vi "Create Counter Driven Output Module.vi"(8 "error in":errorcluster, 9 "channel settings":T2[](array[typedef]), 10 "drive from slot":T1, 11 "module in":refnum<class "Module.lvclass">) -> (0 "error out":errorcluster, 3 "module out":refnum<class "Module.lvclass">)   [LabVIEW 2017, in "Scan Engine Scripting.lvlib" / "Module.lvclass"]
uses:
  Module.lvclass
  Mode Classes/Controls/counter driven output channel settings.ctl
  Channel Classes/Counter Driven Output Channel/Counter Driven State.ctl
  Mode Classes/Counter Driven Output Mode/Drive from Slot.ctl
  Mode Classes/Counter Driven Output Mode/Counter Driven Output Mode.lvclass
  C:/Users/nitest/Documents/niveristand-scan-engine-ethercat-custom-device/Custom Device Source/Scripting/Modules/Mode Classes/Mode/Mode.lvclass
  Channel Classes/Counter Driven Output Channel/Counter Driven Output Channel.lvclass
  C:/Users/nitest/Documents/niveristand-scan-engine-ethercat-custom-device/Custom Device Source/Scripting/Modules/Channel Classes/Channel/Channel.lvclass
  Scan Engine Scripting.lvlib
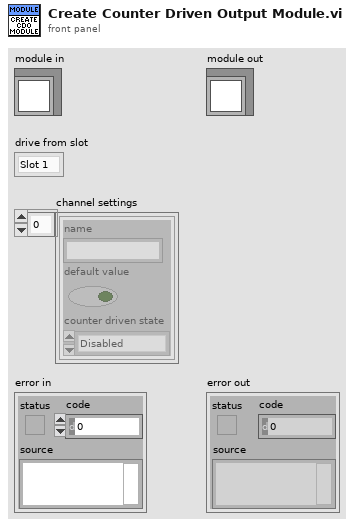
[diagram p1: front panel]
types:
  T1 = typedef "Scan Engine Scripting.lvlib/Counter Driven Output Mode.lvclass/Drive from Slot.ctl" = enum16{"Slot 1", "Slot 2", "Slot 3", "Slot 4", "Slot 5", "Slot 6", "Slot 7", "Slot 8"}
  T2 = typedef "Scan Engine Scripting.lvlib/counter driven output channel settings.ctl" = cluster{"name":string, "default value":bool, "counter driven state":T3}
  T3 = typedef "Scan Engine Scripting.lvlib/Counter Driven Output Channel.lvclass/Counter Driven State.ctl" = enum16{"Disabled", "Enabled"}
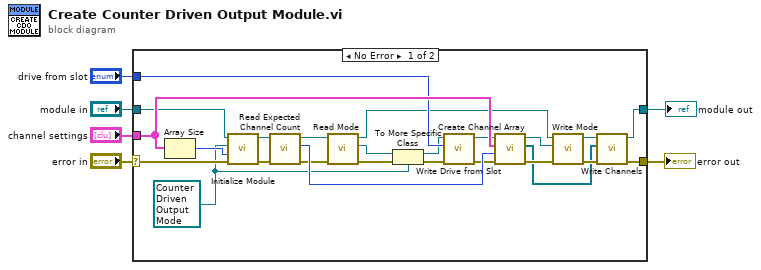
[diagram p0: block diagram]
diagram:
  n1 = case shown="No Error" "error in" {
    selector: "error in" -> [w30 w33]
    tunnel: [w7 w33] -> w1
    tunnel: [w27 w32] -> w2
    tunnel: "module in" -> [w25 w32]
    tunnel: "channel settings" -> [w28 _]
    tunnel: "drive from slot" -> [w24 _]
    frame No Error {
      w17 = refnum<class "Counter Driven Output Mode.lvclass"> refnum ("Scan Engine Scripting.lvlib:Counter Driven Output Mode.lvclass")
      n2 = Array Size(array=w28) -> (size(s)=w21:i32)
      n3 = call-dynamic "Initialize Module.vi"("error in"=w30, "channel array size"=w21, "mode"=w17, "module in"=w25) -> ("error out"=w31:errorcluster, "module out"=w29:refnum<class "Module.lvclass">)  [unwired: 6 in]
      n4 = call-dynamic "Read Expected Channel Count.vi"("error in"=w31, "module in"=w29) -> ("error out"=w20:errorcluster, "expected channel count"=w26:i32, "module out"=w9:refnum<class "Module.lvclass">)  [unwired: 7 in]
      n5 = call-dynamic "Read Mode.vi"("error in"=w20, "module in"=w9) -> ("error out"=w18:errorcluster, "mode"=w19:refnum<class "Mode.lvclass">, "module out"=w8:refnum<class "Module.lvclass">)  [unwired: 7 in]
      n6 = To More Specific Class(target class=w17, reference=w19, error in=w18) -> (specific class reference=w16:refnum<class "Counter Driven Output Mode.lvclass">, error out=w15:errorcluster)
      n7 = call-dynamic "Write Drive from Slot.vi"("error in"=w15, "drive from slot"=w24, "counter driven output mode in"=w16) -> ("error out"=w23:errorcluster, "counter driven output mode out"=w22:refnum<class "Counter Driven Output Mode.lvclass">)  [unwired: 7 in]
      n8 = call "Create Channel Array.vi"("error in"=w23, "array size"=w26, "channel settings"=w28, "counter driven output mode in"=w22) -> ("error out"=w12:errorcluster, "channels"=w10:refnum<class "Counter Driven Output Channel.lvclass">[], "counter driven output mode out"=w13:refnum<class "Counter Driven Output Mode.lvclass">)  [unwired: 5 in]
      n9 = call-dynamic "Write Mode.vi"("error in"=w12, "mode"=w13, "module in"=w8) -> ("error out"=w11:errorcluster, "module out"=w14:refnum<class "Module.lvclass">)  [unwired: 7 in]
      n10 = call-dynamic "Write Channels.vi"("error in"=w11, "channels"=w10, "module in"=w14) -> ("error out"=w7:errorcluster, "module out"=w27:refnum<class "Module.lvclass">)  [unwired: 7 in]
    }
    frame Error {
    }
  }
  "error out" <- w1
  "module out" <- w2
